vi "OpenFile.vi"(8 "error in (no error)":errorcluster, 10 "Nazwa obrazu: 3":string="testowy", 11 "Sciezka:  2":path=path "d:/img") -> (0 "error out":errorcluster, 3 "Image 2":T1(plugin-control))   [LabVIEW 2023]
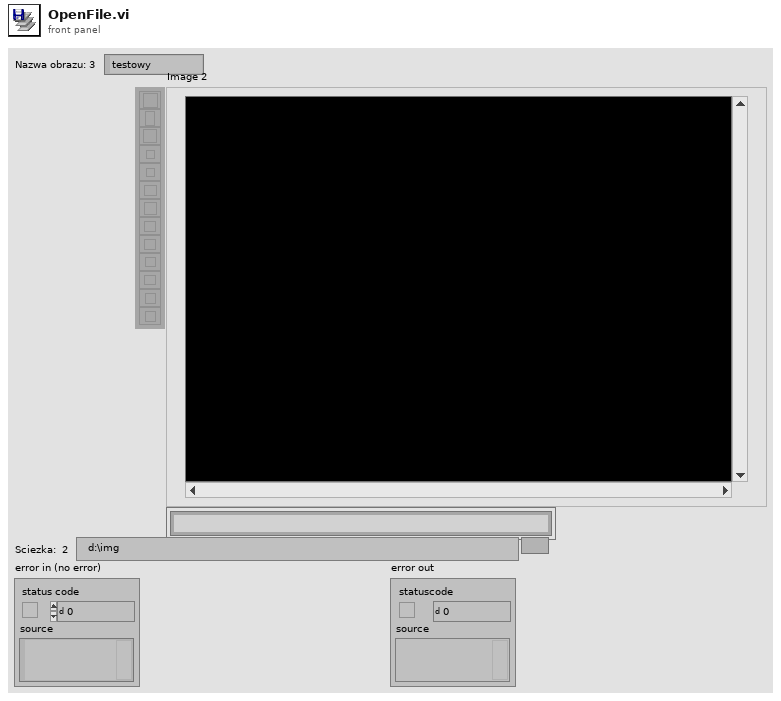
[diagram p1: front panel]
types:
  T1 = typedef "IMAQ Image.ctl" = refnum<image>
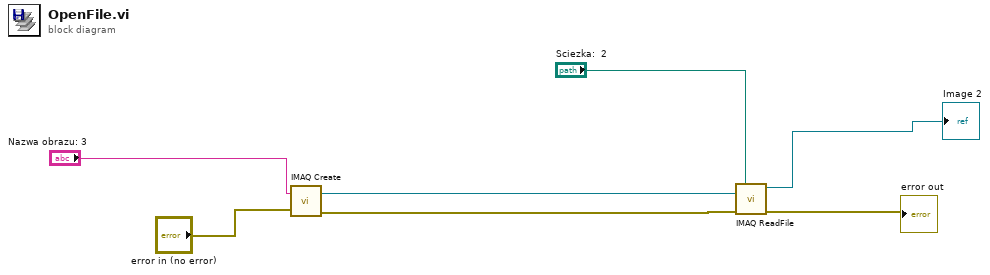
[diagram p0: block diagram]
diagram:
  n1 = call "IMAQ Create"("Image Name"="Nazwa obrazu: 3", "error in (no error)"="error in (no error)") -> ("New Image"=w7:T1, "error out"=w6:errorcluster)  [unwired: 2 in, 1 out]
  n2 = call "IMAQ ReadFile"("File Path"="Sciezka:  2", "error in (no error)"=w6, "Image"=w7) -> ("error out"=→"error out":errorcluster, "Image Out"=→"Image 2":T1)  [unwired: 2 in, 5 out]
